vi "Init Events.vi"(8 "error in (no error)":errorcluster, 11 "Sequencing Control in":refnum<class "Sequencing Control.lvclass">) -> (0 "error out":errorcluster, 3 "Sequencing Control out":refnum<class "Sequencing Control.lvclass">)   [LabVIEW 2020, in "VolatusSeqGUI.lvlib" / "Sequencing Control.lvclass"]
uses:
  Sequencing Control.lvclass
  Sequencing Control.lvclass/Sequencing Control.ctl
  Action.ctl
  Action Data.ctl
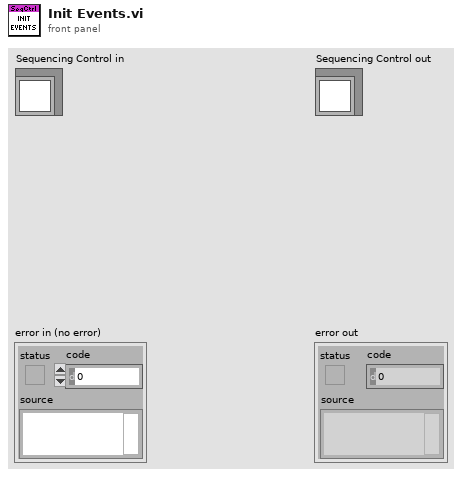
[diagram p1: front panel]
types:
  T1 = typedef "VolatusSeqGUI.lvlib/Sequencing Control.lvclass/Action Data.ctl" = cluster{"Action":T2, "Sequence":string}
  T2 = typedef "VolatusSeqGUI.lvlib/Sequencing Control.lvclass/Action.ctl" = enum16{"Details", "Load", "Unload", "Run", "Abort", "Unload All", "Abort All"}
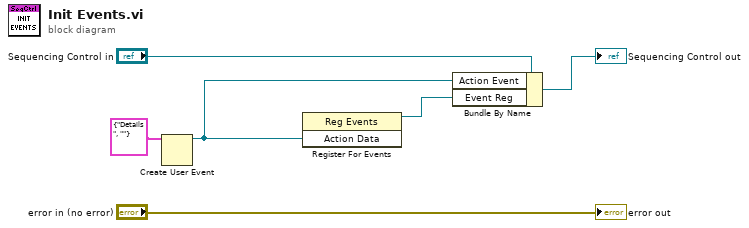
[diagram p0: block diagram]
diagram:
  n1 = Create User Event(user event datatype=T1 {"Action"=enum."Details", "Sequence"=""} ("Action Data")) -> (user event=w1:refnum<user-event>)  [unwired: 1 in, 1 out]
  n2 = register-events(w1) -> (reference out=w2:refnum<event-registration>)  [unwired: 2 in, 1 out]
  n3 = Bundle By Name(cluster="Sequencing Control in", "Action Event"=w1, "Event Reg"=w2) -> (→"Sequencing Control out":refnum<class "Sequencing Control.lvclass">)
  "error out" <- "error in (no error)"
